vi "Pre Loop Init.vi"(8 "error in (no error)":errorcluster) -> (0 "error out":errorcluster)   [LabVIEW 2019]
doc: "Este VI ejecuta las acciones de inicialización antes de entrar en el loop."
uses:
  Private Controls/Queue FGV Action.ctl
  Private Controls/Control HMI Data Cluster.ctl
  Private Controls/Estados.ctl
  Prueba04/Prueba04.lvclass
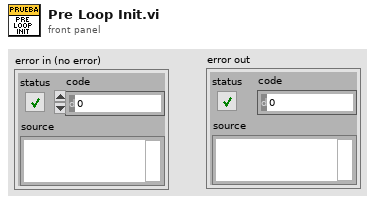
[diagram p1: front panel]
types:
  T1 = typedef "Control HMI Data Cluster.ctl" = cluster{"Estados":T2, "Data":variant}
  T2 = typedef "Estados.ctl" = enum16{"CargaReferencias", "LeerArchivoConfiguracion", "RevisaTipoGenerador", "inicio", "conf_instru", "escribe_frec", "lee_BD", "lee_referencia", "guardarVrefA", "guardarVrefC", "guardarVrefZ", "FrecAmp_A1", "FrecAmp_C1", "FrecAmp_Z1", "FrecAmp_A2", "FrecAmp_C2", "FrecAmp_Z2", "iniciarGEN", "monitoreo", "detenerGEN", "crea_voltajes_prueba_A", "crea_voltajes_prueba_C", "crea_voltajes_prueba_Z", "voltajeInicialA2", "voltajeInicialC2", "voltajeInicialZ2", "actualizarVrefA", "actualizarVrefC", "actualizarVrefZ", "ingresaMedicionesA", "ingresaMedicionesC", "ingresaMedicionesZ", "cumplimiento", "listo_evaluar", "evaluar", "final", "guardaMedicionesA", "guardaMedicionesC", "guardaMedicionesZ", "ultimaFrec", "generaA2", "detieneA2", "salir", "Error"}
  T3 = typedef "Queue FGV Action.ctl" = enum16{"Set", "Get", "Release"}
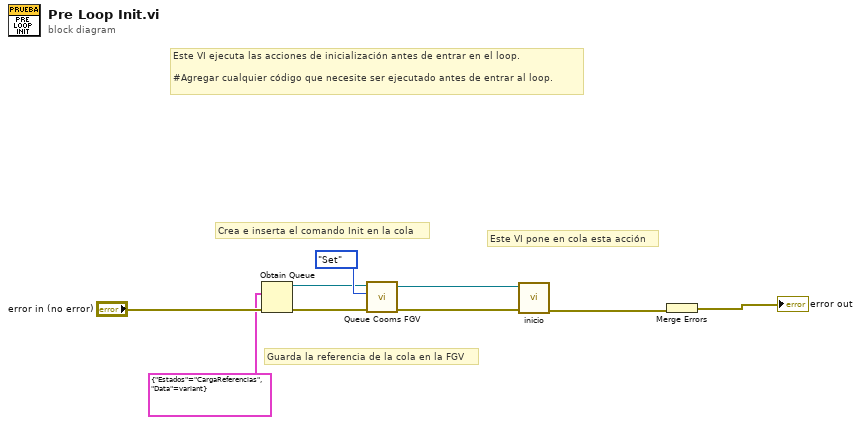
[diagram p0: block diagram]
diagram:
  # "Este VI pone en cola esta acción"
  # "Crea e inserta el comando Init en la cola"
  # "Este VI ejecuta las acciones de inicialización antes de entrar en el loop.\n\n#Agregar cualquier código que necesite ser ejecutado antes de entrar al loop."
  # "Guarda la referencia de la cola en la FGV"
  n1 = Obtain Queue(element data type=T1 {"Estados"=enum."CargaReferencias", "Data"=variant} ("Module Dat Cluster"), error in (no error)="error in (no error)") -> (queue out=w3:refnum<queue>, error out=w9:errorcluster)  [unwired: 3 in, 1 out]
  n2 = call "Queue Cooms FGV.vi"("error in"=w9, "Action"=Queue_FGV_Action."Set", "queue in"=w3) -> ("error out"=w5:errorcluster, "queue out"=w2:refnum<queue>)  [unwired: 7 in]
  n3 = call "inicio.vi"("error in (no error)"=w5, "Data"=w2) -> ("error out"=w4:errorcluster)  [unwired: 9 in]
  n4 = Merge Errors(w4) -> (→"error out":errorcluster)
